vi "Get Hough Lines.vi"(4 "Error":string, 5 "Input Hough":T1=[{"r"=0.0, "q"=-1, "count"=0}, {"r"=0.0, "q"=-1, "count"=0}, {"r"=0.0, "q"=-1, "count"=0}, {"r"=0.0, "q"=-1, "count"=0}, {"r"=0.0, "q"=-1, "count"=0}, {"r"=0.0, "q"=-1, "count"=0}, {"r"=1.0, "q"=-1, "count"=0}, {"r"=0.0, "q"=-1, "count"=0}, {"r"=0.0, "q"=-1, "count"=0}, {"r"=0.0, "q"=-1, "count"=0}, {"r"=0.0, "q"=-1, "count"=0}, {"r"=0.0, "q"=-1, "count"=0}, {"r"=0.0, "q"=-1, "count"=0}, {"r"=0.0, "q"=-1, "count"=0}, {"r"=0.0, "q"=-1, "count"=0}, {"r"=0.0, "q"=-1, "count"=0}, {"r"=0.0, "q"=-1, "count"=0}, {"r"=0.0, "q"=-1, "count"=0}, {"r"=0.0, "q"=-1, "count"=0}, {"r"=0.0, "q"=-1, "count"=0}, {"r"=0.0, "q"=-1, "count"=0}, {"r"=0.0, "q"=-1, "count"=0}, {"r"=0.0, "q"=-1, "count"=0}, {"r"=0.0, "q"=-1, "count"=0}, {"r"=0.0, "q"=-1, "count"=0}, {"r"=0.0, "q"=-1, "count"=0}, {"r"=0.0, "q"=-1, "count"=0}, {"r"=0.0, "q"=-1, "count"=0}, {"r"=0.0, "q"=-1, "count"=0}, {"r"=0.0, "q"=-1, "count"=0}, {"r"=0.0, "q"=-1, "count"=0}, {"r"=0.0, "q"=-1, "count"=0}, {"r"=0.0, "q"=-1, "count"=0}, {"r"=0.0, "q"=-1, "count"=0}, {"r"=0.0, "q"=-1, "count"=0}, {"r"=0.0, "q"=-1, "count"=0}, {"r"=0.0, "q"=-1, "count"=0}, {"r"=0.0, "q"=-1, "count"=0}, {"r"=0.0, "q"=-1, "count"=0}, {"r"=0.0, "q"=-1, "count"=0}, {"r"=0.0, "q"=-1, "count"=0}, {"r"=0.0, "q"=-1, "count"=0}, {"r"=0.0, "q"=-1, "count"=0}, {"r"=0.0, "q"=-1, "count"=0}, {"r"=0.0, "q"=-1, "count"=0}, {"r"=0.0, "q"=-1, "count"=0}, {"r"=0.0, "q"=-1, "count"=0}, {"r"=0.0, "q"=-1, "count"=0}, {"r"=0.0, "q"=-1, "count"=0}, {"r"=0.0, "q"=-1, "count"=0}, {"r"=0.0, "q"=-1, "count"=0}, {"r"=0.0, "q"=-1, "count"=0}, {"r"=0.0, "q"=-1, "count"=0}, {"r"=0.0, "q"=-1, "count"=0}, {"r"=0.0, "q"=-1, "count"=0}, {"r"=0.0, "q"=-1, "count"=0}, {"r"=0.0, "q"=-1, "count"=0}, {"r"=0.0, "q"=-1, "count"=0}, {"r"=0.0, "q"=-1, "count"=0}, {"r"=0.0, "q"=-1, "count"=0}, {"r"=0.0, "q"=-1, "count"=0}, {"r"=0.0, "q"=-1, "count"=0}, {"r"=0.0, "q"=-1, "count"=0}, {"r"=0.0, "q"=-1, "count"=0}, {"r"=0.0, "q"=-1, "count"=0}, {"r"=0.0, "q"=-1, "count"=0}, {"r"=0.0, "q"=-1, "count"=0}, {"r"=0.0, "q"=-1, "count"=0}, {"r"=0.0, "q"=-1, "count"=0}, {"r"=0.0, "q"=-1, "count"=0}, {"r"=0.0, "q"=-1, "count"=0}, {"r"=0.0, "q"=-1, "count"=0}, {"r"=0.0, "q"=-1, "count"=0}, {"r"=0.0, "q"=-1, "count"=0}, {"r"=0.0, "q"=-1, "count"=0}, {"r"=0.0, "q"=-1, "count"=0}, {"r"=0.0, "q"=-1, "count"=0}, {"r"=0.0, "q"=-1, "count"=0}, {"r"=0.0, "q"=-1, "count"=0}, {"r"=0.0, "q"=-1, "count"=0}, {"r"=0.0, "q"=-1, "count"=0}, {"r"=0.0, "q"=-1, "count"=0}, {"r"=0.0, "q"=-1, "count"=0}, {"r"=0.0, "q"=-1, "count"=0}, {"r"=0.0, "q"=-1, "count"=0}, {"r"=0.0, "q"=-1, "count"=0}, {"r"=0.0, "q"=-1, "count"=0}, {"r"=0.0, "q"=-1, "count"=0}, {"r"=0.0, "q"=-1, "count"=0}, {"r"=0.0, "q"=-1, "count"=0}, {"r"=0.0, "q"=-1, "count"=0}, {"r"=0.0, "q"=-1, "count"=0}, {"r"=0.0, "q"=-1, "count"=0}, {"r"=0.0, "q"=-1, "count"=0}, {"r"=0.0, "q"=-1, "count"=0}, {"r"=0.0, "q"=-1, "count"=0}, {"r"=0.0, "q"=-1, "count"=0}, {"r"=0.0, "q"=-1, "count"=0}, {"r"=0.0, "q"=-1, "count"=0}, {"r"=0.0, "q"=-1, "count"=0}, {"r"=0.0, "q"=-1, "count"=0}, {"r"=0.0, "q"=-1, "count"=0}, {"r"=0.0, "q"=-1, "count"=0}, {"r"=0.0, "q"=-1, "count"=0}, {"r"=0.0, "q"=-1, "count"=0}, {"r"=0.0, "q"=-1, "count"=0}, {"r"=0.0, "q"=-1, "count"=0}, {"r"=0.0, "q"=-1, "count"=0}, {"r"=0.0, "q"=-1, "count"=0}, {"r"=0.0, "q"=-1, "count"=0}, {"r"=0.0, "q"=-1, "count"=0}, {"r"=0.0, "q"=-1, "count"=0}, {"r"=0.0, "q"=-1, "count"=0}, {"r"=0.0, "q"=-1, "count"=0}, {"r"=0.0, "q"=-1, "count"=0}, {"r"=0.0, "q"=-1, "count"=0}, {"r"=0.0, "q"=-1, "count"=0}, {"r"=0.0, "q"=-1, "count"=0}, {"r"=0.0, "q"=-1, "count"=0}, {"r"=0.0, "q"=-1, "count"=0}, {"r"=0.0, "q"=-1, "count"=0}, {"r"=0.0, "q"=-1, "count"=0}, {"r"=0.0, "q"=-1, "count"=0}, {"r"=0.0, "q"=-1, "count"=0}, {"r"=0.0, "q"=-1, "count"=0}, {"r"=0.0, "q"=-1, "count"=0}, {"r"=0.0, "q"=-1, "count"=0}, {"r"=0.0, "q"=-1, "count"=0}, {"r"=0.0, "q"=-1, "count"=0}, {"r"=0.0, "q"=-1, "count"=0}, {"r"=0.0, "q"=-1, "count"=0}, {"r"=0.0, "q"=-1, "count"=0}, {"r"=0.0, "q"=-1, "count"=0}, {"r"=0.0, "q"=-1, "count"=0}, {"r"=0.0, "q"=-1, "count"=0}, {"r"=0.0, "q"=-1, "count"=0}, {"r"=0.0, "q"=-1, "count"=0}, {"r"=0.0, "q"=-1, "count"=0}, {"r"=0.0, "q"=-1, "count"=0}, {"r"=0.0, "q"=-1, "count"=0}, {"r"=0.0, "q"=-1, "count"=0}, {"r"=0.0, "q"=-1, "count"=0}, {"r"=0.0, "q"=-1, "count"=0}, {"r"=0.0, "q"=-1, "count"=0}, {"r"=0.0, "q"=-1, "count"=0}, {"r"=0.0, "q"=-1, "count"=0}, {"r"=0.0, "q"=-1, "count"=0}, {"r"=0.0, "q"=-1, "count"=0}, {"r"=0.0, "q"=-1, "count"=0}, {"r"=0.0, "q"=-1, "count"=0}, {"r"=0.0, "q"=-1, "count"=0}, {"r"=0.0, "q"=-1, "count"=0}, {"r"=0.0, "q"=-1, "count"=0}, {"r"=0.0, "q"=-1, "count"=0}, {"r"=0.0, "q"=-1, "count"=0}, {"r"=0.0, "q"=-1, "count"=0}, {"r"=0.0, "q"=-1, "count"=0}, {"r"=0.0, "q"=-1, "count"=0}, {"r"=0.0, "q"=-1, "count"=0}, {"r"=0.0, "q"=-1, "count"=0}, {"r"=0.0, "q"=-1, "count"=0}, {"r"=0.0, "q"=-1, "count"=0}, {"r"=0.0, "q"=-1, "count"=0}, {"r"=0.0, "q"=-1, "count"=0}, {"r"=0.0, "q"=-1, "count"=0}, {"r"=0.0, "q"=-1, "count"=0}, {"r"=0.0, "q"=-1, "count"=0}, {"r"=0.0, "q"=-1, "count"=0}, {"r"=0.0, "q"=-1, "count"=0}, {"r"=0.0, "q"=-1, "count"=0}, {"r"=0.0, "q"=-1, "count"=0}, {"r"=0.0, "q"=-1, "count"=0}, {"r"=0.0, "q"=-1, "count"=0}, {"r"=0.0, "q"=-1, "count"=0}, {"r"=0.0, "q"=-1, "count"=0}, {"r"=0.0, "q"=-1, "count"=0}, {"r"=0.0, "q"=-1, "count"=0}, {"r"=0.0, "q"=-1, "count"=0}, {"r"=0.0, "q"=-1, "count"=0}, {"r"=0.0, "q"=-1, "count"=0}, {"r"=0.0, "q"=-1, "count"=0}, {"r"=0.0, "q"=-1, "count"=0}, {"r"=0.0, "q"=-1, "count"=0}, {"r"=0.0, "q"=-1, "count"=0}, {"r"=0.0, "q"=-1, "count"=0}, {"r"=0.0, "q"=-1, "count"=0}, {"r"=0.0, "q"=-1, "count"=0}, {"r"=0.0, "q"=-1, "count"=0}, {"r"=0.0, "q"=-1, "count"=0}, {"r"=0.0, "q"=-1, "count"=0}, {"r"=0.0, "q"=-1, "count"=0}, {"r"=0.0, "q"=-1, "count"=0}, {"r"=0.0, "q"=-1, "count"=0}, {"r"=0.0, "q"=-1, "count"=0}, {"r"=0.0, "q"=-1, "count"=0}, {"r"=0.0, "q"=-1, "count"=0}, {"r"=0.0, "q"=-1, "count"=0}, {"r"=0.0, "q"=-1, "count"=0}, {"r"=0.0, "q"=-1, "count"=0}, {"r"=0.0, "q"=-1, "count"=0}, {"r"=0.0, "q"=-1, "count"=0}], 6 "Threshold":u16, 7 "Hough's Transform's Result":i16) -> (0 "Error":string, 1 "Output Lines":T1, 2 "Total Number of Lines":u16, 3 "Hough's Transform's Result":i16)   [LabVIEW 2011, in "labvvis.lvlib"]
doc: "Returns an array with 256 elements, where each element in the array contains the number of times pixels equal to the index is encountered in Input Image.\n\nIf you connect an array that does not have 256 elements, this VI will not execute. If you do not connect an array at all, this VI will provide one.\n\nNote that this VI only operates on single-channel images. Thus grey-scale, Red channel, Green channel and so on images are supported. RGBA images are not supported."
uses:
  <userlib>/labvvis/labvvis.lvlib
  <userlib>/labvvis/Many Hough Lines.ctl
  <userlib>/labvvis/Hough Line.ctl
  labvvis.framework
panel:
  out "Threshold":u16
  in  "Total Number of Lines":u16
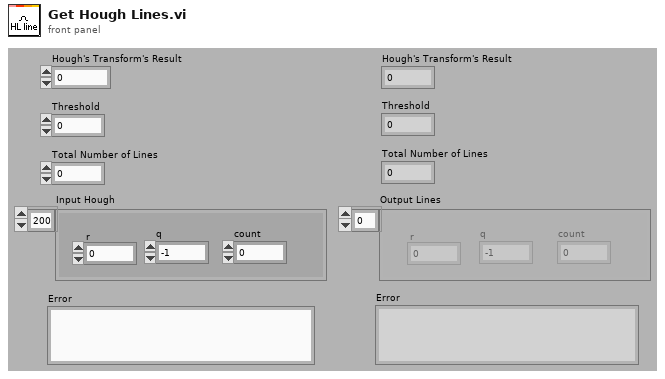
[diagram p1: front panel]
types:
  T1 = typedef "labvvis.lvlib/Many Hough Lines.ctl" = T2[]
  T2 = typedef "labvvis.lvlib/Hough Line.ctl" = cluster{"r":dbl, "q":i16, "count":i16}
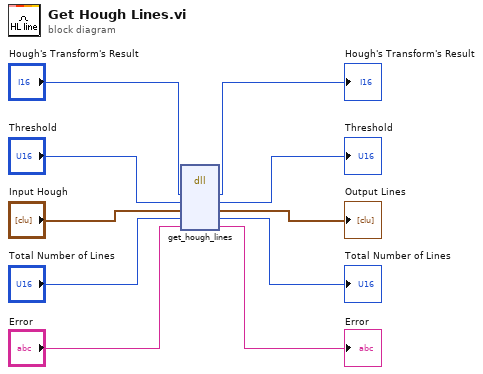
[diagram p0: block diagram]
diagram:
  n1 = dll-call lib="labvvis.framework" fn="get_hough_lines"("hough_id"="Hough's Transform's Result", "threshold"="Threshold", "Input Hough"="Input Hough", "lines_count"="Total Number of Lines", "error"="Error") -> ("hough_id"=→"Hough's Transform's Result":i16, "threshold"=→"Threshold":u16, "Input Hough"=→"Output Lines":T1, "lines_count"=→"Total Number of Lines":u16, "error"=→"Error":string)  [unwired: 4 in, 2 out]
